vi "Read PID.vi"(8 "error in (no error)":errorcluster, 11 "PIDController in":refnum<class "PIDController.lvclass">) -> (0 "error out":errorcluster, 2 "register values":dbl[](array[numeric]), 3 "PIDController out":refnum<class "PIDController.lvclass">)   [LabVIEW 2023, in "PIDController.lvclass"]
uses:
  PIDController.lvclass
  PIDController.lvclass/PIDController.ctl
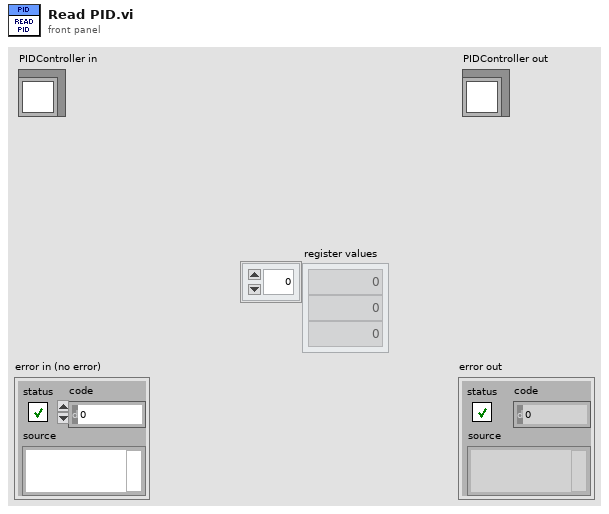
[diagram p1: front panel]
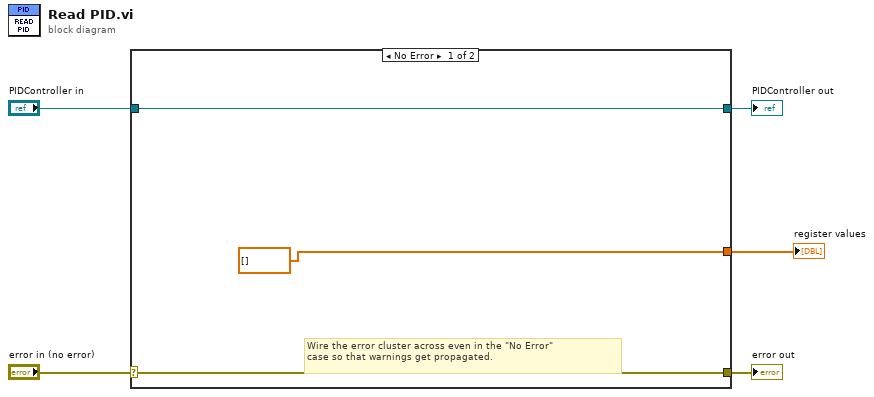
[diagram p0: block diagram]
diagram:
  n1 = case shown="No Error" "error in (no error)" {
    selector: "error in (no error)" -> [w7 w10]
    tunnel: [w7 w10] -> w4
    tunnel: [w8 w9] -> w2
    tunnel: "PIDController in" -> [w8 w9]
    tunnel: [dbl[] [] ("register values") _] -> w1
    frame No Error {
      # "Wire the error cluster across even in the \"No Error\"\ncase so that warnings get propagated."
    }
    frame Error {
    }
  }
  "error out" <- w4
  "PIDController out" <- w2
  "register values" <- w1
